vi "Plot.vi"(8 "error in (no error)":errorcluster, 11 "Electrometer.lvclass":refnum<class "Electrometer.lvclass">) -> (0 "error out":errorcluster)   [LabVIEW 2016]
uses:
  Electrometer/Electrometer.lvclass
panel:
  out "Measurement":dbl(graph)
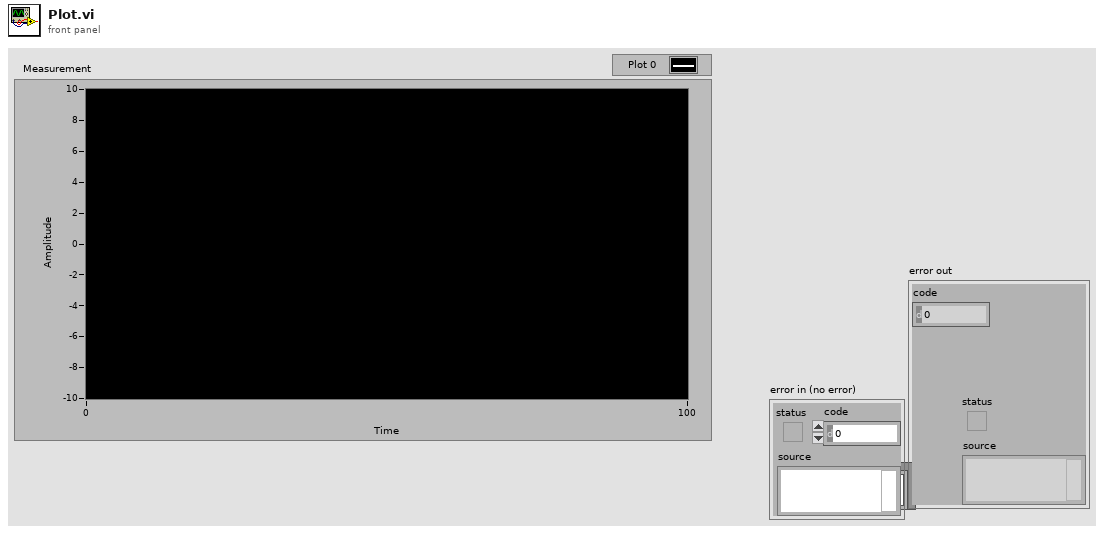
[diagram p1: front panel]
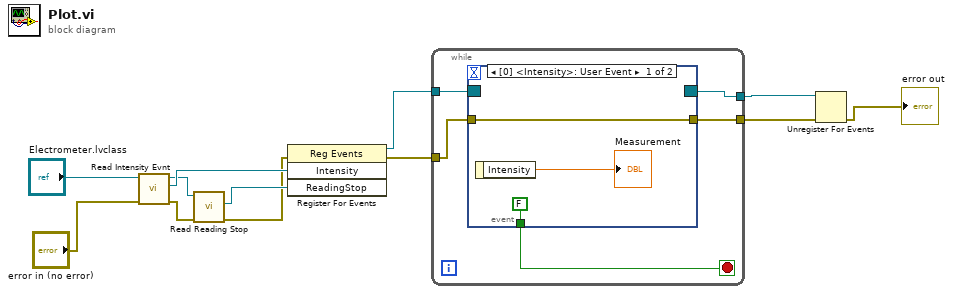
[diagram p0: block diagram]
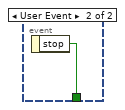
[diagram p2: hidden frame]
diagram:
  n1 = call-dynamic "Read Intensity Evnt.vi"("error in (no error)"="error in (no error)", "Electrometer in"="Electrometer.lvclass") -> ("error out"=w4:errorcluster, "Intensity"=w11:refnum<user-event>, "Electrometer out"=w3:refnum<class "Electrometer.lvclass">)  [unwired: 7 in]
  n2 = call-dynamic "Read Reading Stop.vi"("error in (no error)"=w4, "Electrometer in"=w3) -> ("error out"=w1:errorcluster, "ReadingStop"=w2:refnum<user-event>)  [unwired: 7 in, 1 out]
  n3 = register-events(error in=w1, w11, w2) -> (reference out=w10:refnum<event-registration>, error out=w8:errorcluster)  [unwired: 1 in]
  n4 = while {
    tunnel: w10 -> [w17]
    tunnel: w8 -> [w14]
    tunnel: [w16] -> w7
    tunnel: [w15] -> w5
    stop <- w13 stop-if-true
    n5 = event shown="[0] <Intensity>: User Event" {
      selector: w17 -> [_ _]
      dyn-events: [_ _] -> w16
      timeout: _ -> [_ _]
      tunnel: [w19 _] -> w15
      tunnel: w14 -> [w19 _]
      tunnel: [FALSE ("stop") w21] -> w13
      event User Event {
        n6 = event-data() -> ("Intensity"=→"Measurement":dbl)  [unwired: 1 in]
      }
      event User Event {
        n7 = event-data() -> ("stop"=w21:bool)  [unwired: 1 in]
      }
    }
  }
  n8 = Unregister For Events(event registration refnum=w7, error in=w5) -> (error out=→"error out":errorcluster)
